vi "Periodic - Shooter PID Loop.vi"() -> ()   [LabVIEW 2012]
uses:
  Globals/Jaguar Commands.vi
  Globals/Encoders Global.vi
  Globals/Shooter Speed Error.vi
panel:
  out "Error":dbl
  out "Shooter Speed Error":dbl(knob) scale=-200.0..200.0
  in  "PID gains (Shooter)":T1={"proportional gain (Kc)"=30.0, "integral time (Ti, min)"=0.0, "derivative time (Td, min)"=0.0} {"proportional gain (Kc)" format="%.6g"; "integral time (Ti, min)" format="%.6g"; "derivative time (Td, min)" format="%.6g"}
  in  "Inverted?":bool=TRUE
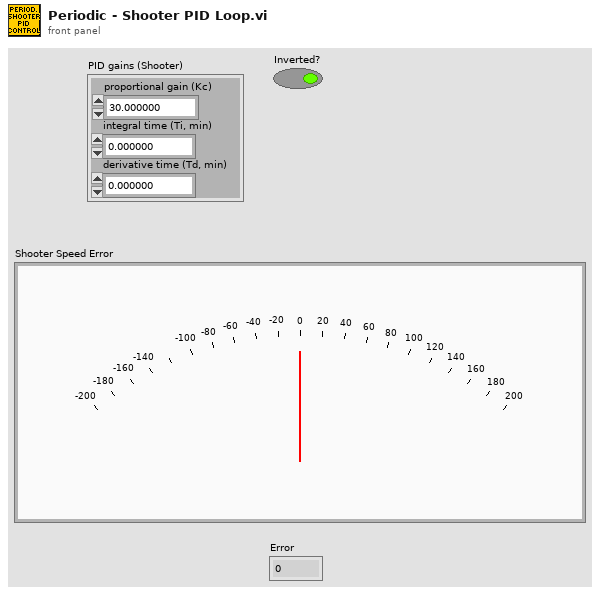
[diagram p1: front panel]
types:
  T1 = cluster{"proportional gain (Kc)":dbl, "integral time (Ti, min)":dbl, "derivative time (Td, min)":dbl}
  T2 = typedef "WPI_EncoderDevRef.ctl" = cluster{"DevStatus":errorcluster, "EncoderIndex":T3, "CounterIndex":T4, "DistancePerCount":dbl, "Decoding Type":T5}
  T3 = typedef "FPGA_EncoderIdx.ctl" = enum8{"Enc 0", "Enc 1", "Enc 2", "Enc 3", "Invalid"}
  T4 = typedef "FPGA_CounterCtrSystemIndex.ctl" = enum8{"Ctr 0", "Ctr 1", "Ctr 2", "Ctr 3", "Ctr 4", "Ctr 5", "Ctr 6", "Ctr 7", "Invalid"}
  T5 = typedef "WPI_EncoderType.ctl" = enum16{"1x", "2x", "4x"}
  T6 = cluster{"Front Left":T2, "Front Right":T2, "Rear Left":T2, "Rear Right":T2, "Shooter":T2}
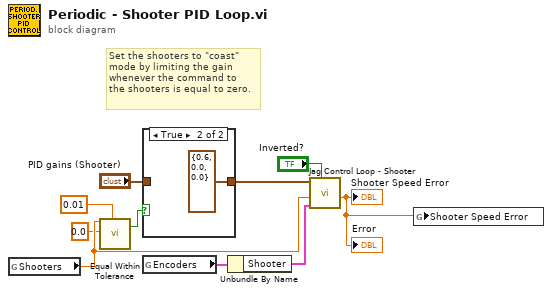
[diagram p0: block diagram]
diagram:
  # "Set the shooters to \"coast\"\nmode by limiting the gain\nwhenever the command to\nthe shooters is equal to zero."
  n1 = global read "Jaguar Commands.vi" "Shooters"() -> (w10:dbl)
  n2 = call "Equal Within Tolerance.vi"("Number In"=w10, "Comparison Value"=0.0, "Tolerance"=0.01) -> ("Equality"=w2:bool)  [unwired: 16 in]
  n3 = case shown="True" w2 {
    tunnel: "PID gains (Shooter)" -> [w11 _]
    tunnel: [w11 T1 {"proportional gain (Kc)"=0.6, "integral time (Ti, min)"=0.0, "derivative time (Td, min)"=0.0} ("PID gains (Shooter)")] -> w3
    frame False {
    }
    frame True {
    }
  }
  n4 = global read "Encoders Global.vi" "Encoders"() -> (w7:T6)
  n5 = Unbundle By Name(w7) -> ("Shooter"=w9:T2)
  n6 = call "Jag Control Loop - Shooter.vi"("PID gains"=w3, "Command"=w10, "EncoderDevRef"=w9, "Inverted?"="Inverted?") -> ("Error"=w1:dbl)  [unwired: 6 in]
  "Shooter Speed Error" <- w1
  "Error" <- w1
  n7 = global write "Shooter Speed Error.vi" "Shooter Speed Error"(w1) -> ()
